vi "raw data typedef container.vi"() -> (0 "Acquired Data":T1)   [LabVIEW 2019, in "Main.lvclass"]
doc: "Developed by Kevin Thompson\nkevin@thompsonengineering.net\n\nCopyright 2020\nThompson Engineering, LLC"
uses:
  Main.lvclass
  DataTypes/raw data variables.ctl
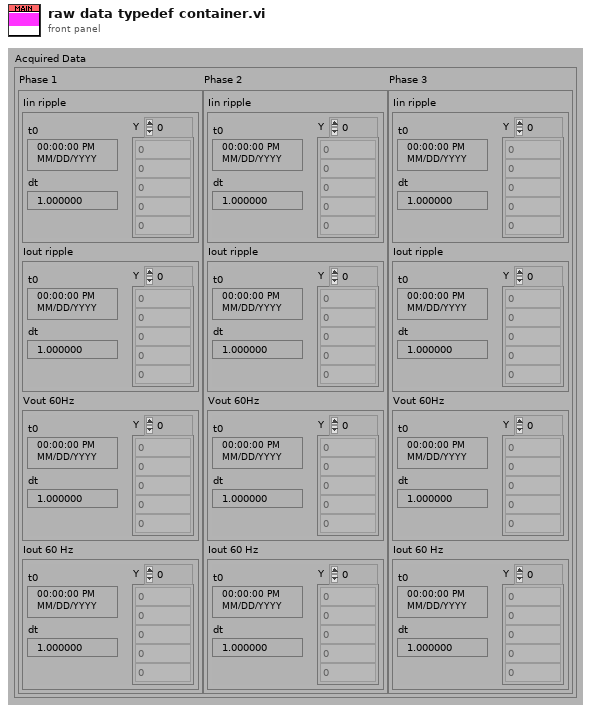
[diagram p1: front panel]
types:
  T1 = typedef "Main.lvclass/raw data variables.ctl" = cluster{"Phase 1":cluster{"Iin ripple":waveform(dbl), "Iout ripple":waveform(dbl), "Vout 60Hz":waveform(dbl), "Iout 60 Hz":waveform(dbl)}, "Phase 2":cluster{"Iin ripple":waveform(dbl), "Iout ripple":waveform(dbl), "Vout 60Hz":waveform(dbl), "Iout 60 Hz":waveform(dbl)}, "Phase 3":cluster{"Iin ripple":waveform(dbl), "Iout ripple":waveform(dbl), "Vout 60Hz":waveform(dbl), "Iout 60 Hz":waveform(dbl)}}
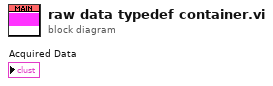
[diagram p0: block diagram]
diagram:
